vi "FRCts20_Backend_INI_Initialize.vi"(6 "Inhibit (F)":bool, 8 "error in (no error)":errorcluster, 10 "Config Path":path=path "C:/Users/Public/Documents/frctsappdata", 11 "INI Controller in":refnum<class "FRCts20_Backend_INI Controller.lvclass">) -> (0 "error out":errorcluster, 3 "INI Controller out":refnum<class "FRCts20_Backend_INI Controller.lvclass">)   [LabVIEW 2014, in "FRCts20_Backend_Engine.lvlib" / "FRCts20_Backend_INI Controller.lvclass"]
uses:
  FRCts20_Backend_INI Controller.lvclass
  FRCts20_Backend_INI Controller.lvclass/FRCts20_Backend_INI Controller.ctl
  <vilib>/Utility/config.llb/NI_LVConfig.lvlib
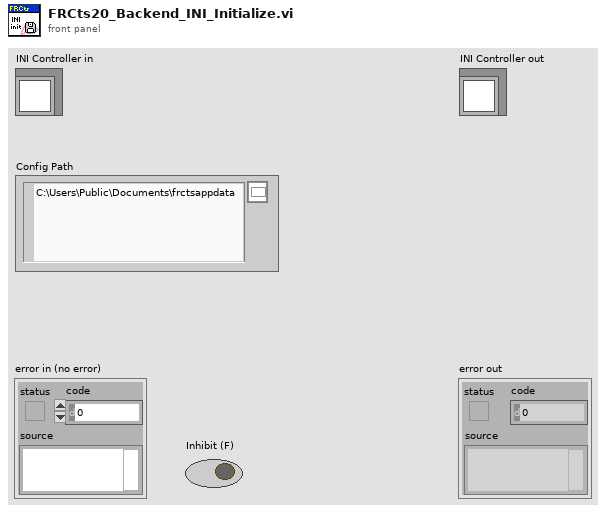
[diagram p1: front panel]
types:
  T1 = typedef "NI_LVConfig.lvlib/Config Data RefNum.ctl" = refnum<k1>
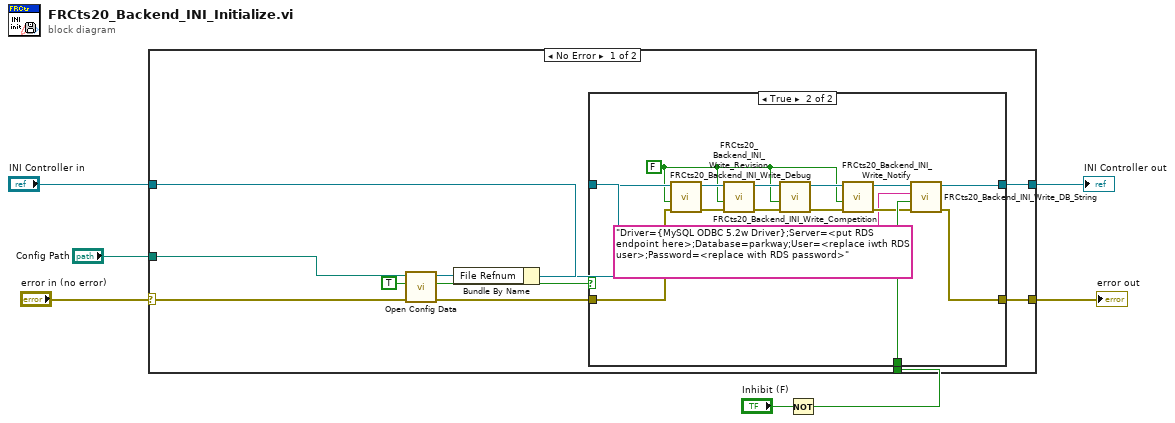
[diagram p0: block diagram]
diagram:
  n1 = Not(x="Inhibit (F)") -> (.not. x?=w1:bool)
  n2 = case shown="No Error" "error in (no error)" {
    selector: "error in (no error)" -> [w17 w37]
    tunnel: [w11 w37] -> w6
    tunnel: [w9 w36] -> w4
    tunnel: "INI Controller in" -> [w16 w36]
    tunnel: "Config Path" -> [w18 _]
    tunnel: w1 -> [w10 _]
    frame No Error {
      n3 = call <vilib>:"Open Config Data.vi"("error in (no error)"=w17, "create file if necessary (T)"=TRUE, "configuration file path"=w18) -> ("error out"=w12:errorcluster, "file created?"=w14:bool, "refnum"=w15:T1)  [unwired: 6 in]
      n4 = Bundle By Name(cluster=w16, "File Refnum"=w15) -> (w13:refnum<class "FRCts20_Backend_INI Controller.lvclass">)
      n5 = case shown="True" w14 {
        tunnel: w13 -> [w20 w35]
        tunnel: w12 -> [w19 w34]
        tunnel: [w20 w31] -> w9
        tunnel: [w19 w29] -> w11
        tunnel: w10 -> [_ w30]
        frame False {
        }
        frame True {
          w22 = FALSE ("Save? (T)")
          n6 = call "FRCts20_Backend_INI_Write_Debug.vi"("error in (no error)"=w34, "Save? (T)"=w22, "INI Controller in"=w35) -> ("error out"=w32:errorcluster, "INI Controller out"=w33:refnum<class "FRCts20_Backend_INI Controller.lvclass">)  [unwired: 7 in]
          n7 = call "FRCts20_Backend_INI_Write_Revision.vi"("error in (no error)"=w32, "Save? (T)"=w22, "INI Controller in"=w33) -> ("error out"=w28:errorcluster, "INI Controller out"=w27:refnum<class "FRCts20_Backend_INI Controller.lvclass">)  [unwired: 7 in]
          n8 = call "FRCts20_Backend_INI_Write_Competition.vi"("error in (no error)"=w28, "Save? (T)"=w22, "INI Controller in"=w27) -> ("error out"=w26:errorcluster, "INI Controller out"=w25:refnum<class "FRCts20_Backend_INI Controller.lvclass">)  [unwired: 7 in]
          n9 = call "FRCts20_Backend_INI_Write_Notify.vi"("error in (no error)"=w26, "Save? (T)"=w22, "INI Controller in"=w25) -> ("error out"=w23:errorcluster, "INI Controller out"=w24:refnum<class "FRCts20_Backend_INI Controller.lvclass">)  [unwired: 7 in]
          n10 = call "FRCts20_Backend_INI_Write_DB_String.vi"("error in (no error)"=w23, "Save? (T)"=w30, "Connection String"="Driver={MySQL ODBC 5.2w Driver};Server=<put RDS endpoint here>;Database=parkway;User=<replace iwth RDS user>;Password=<replace with RDS password>", "INI Controller in"=w24) -> ("error out"=w29:errorcluster, "INI Controller out"=w31:refnum<class "FRCts20_Backend_INI Controller.lvclass">)  [unwired: 6 in]
        }
      }
    }
    frame Error {
    }
  }
  "error out" <- w6
  "INI Controller out" <- w4
